vi "Dual_image_synced_pread.vi"() -> ()   [LabVIEW 2013]
uses:
  <vilib>/vision/driver/NI_Vision_Acquisition_Software.lvlib
  <resource>/objmgr/imaqdx.rc
  <resource>/objmgr/daqmx.rc
  <vilib>/DAQmx/configure/timing.llb/DAQmx Timing (Implicit).vi
  <vilib>/DAQmx/create/channels.llb/DAQmx Create Channel (CO-Pulse Generation-Frequency).vi
  <vilib>/DAQmx/create/channels.llb/DAQmx Create Channel (AO-Voltage-Basic).vi
  <vilib>/DAQmx/write.llb/DAQmx Write (Analog DBL 1Chan 1Samp).vi
  <vilib>/DAQmx/create/channels.llb/DAQmx Create Channel (AI-Voltage-Basic).vi
panel:
  in  "File Location":path=path "C:/Users/Public/Documents/Users_2012_2013/Ryan Gergely/ptest/20150925_Accumulator_trials"
  in  "File Name":string="test"
  in  "stop":bool
  out "Pressure Reading":cluster{dbl[], dbl[]}(graph)
  in  "Pressure Offset":dbl
  out "Current Pressure (Psi)":dbl format="%#_4g"
  in  "Sample Frequency (Hz)":dbl=10.0
  in  "Begin Measurement":bool
  in  "Gain 2":dbl(slide)=575.0 min=350.0 max=1000.0 step=1.0 scale=350.0..1000.0
  in  "VR2":dbl(slide)=65.0 min=0.0 max=255.0 step=1.0 scale=0.0..255.0
  in  "VR1":dbl(slide)=60.0 min=0.0 max=255.0 step=1.0 scale=0.0..255.0
  in  "UB2":dbl(slide)=160.0 min=0.0 max=255.0 step=1.0 scale=0.0..255.0
  in  "UB1":dbl(slide)=165.0 min=0.0 max=255.0 step=1.0 scale=0.0..255.0
  in  "Shutter":dbl(slide)=4095.0 min=0.0 max=4095.0 step=1.0 scale=4.095..4095.0 scale format="%#.0f"
  in  "Brightness":dbl(slide)=100.0 min=0.0 max=255.0 step=1.0 scale=0.0..255.0
  in  "Gain":dbl(slide)=600.0 min=350.0 max=1000.0 step=1.0 scale=350.0..1000.0
  in  "Test Description":string="test"
  in  "Storage Directory":path=path "C:/Users/Regen/Desktop/Users/Ryan Gergely/3D_DIC"
  out "Image 2":T1(plugin-control)
  out "Buffer Number 2":u32
  out "Frame Rate 2":dbl
  in  "Camera Name 2":refnum<k21>="cam2" caption="IMAQdx Session"
  in  "Pule Frequency":dbl=2.0 format="%.1f"
  out "Actual Duty Cycle":dbl
  out "Actual Pulse Frequency":dbl
  in  "Stop":bool
  in  "Start Trigger Mode":bool
  out "Frame Rate 1":dbl
  out "Buffer Number 1":u32
  in  "Camera Name 1":refnum<k21>="cam1" caption="IMAQdx Session"
  out "Image":T1(plugin-control)
  # "1) Set Test Description and Storage Directory"
  # "2) Select Cameras"
  # "3) Start VI"
  # "4) Set Frequency and Exposure and White Balance\n(Before Start Trigger)"
  # "5)"
  # "6) Stop When Done"
  # "Exposure Settings - Both Cameras"
  # "White Balance - Camera1"
  # "White Balance - Camera2"
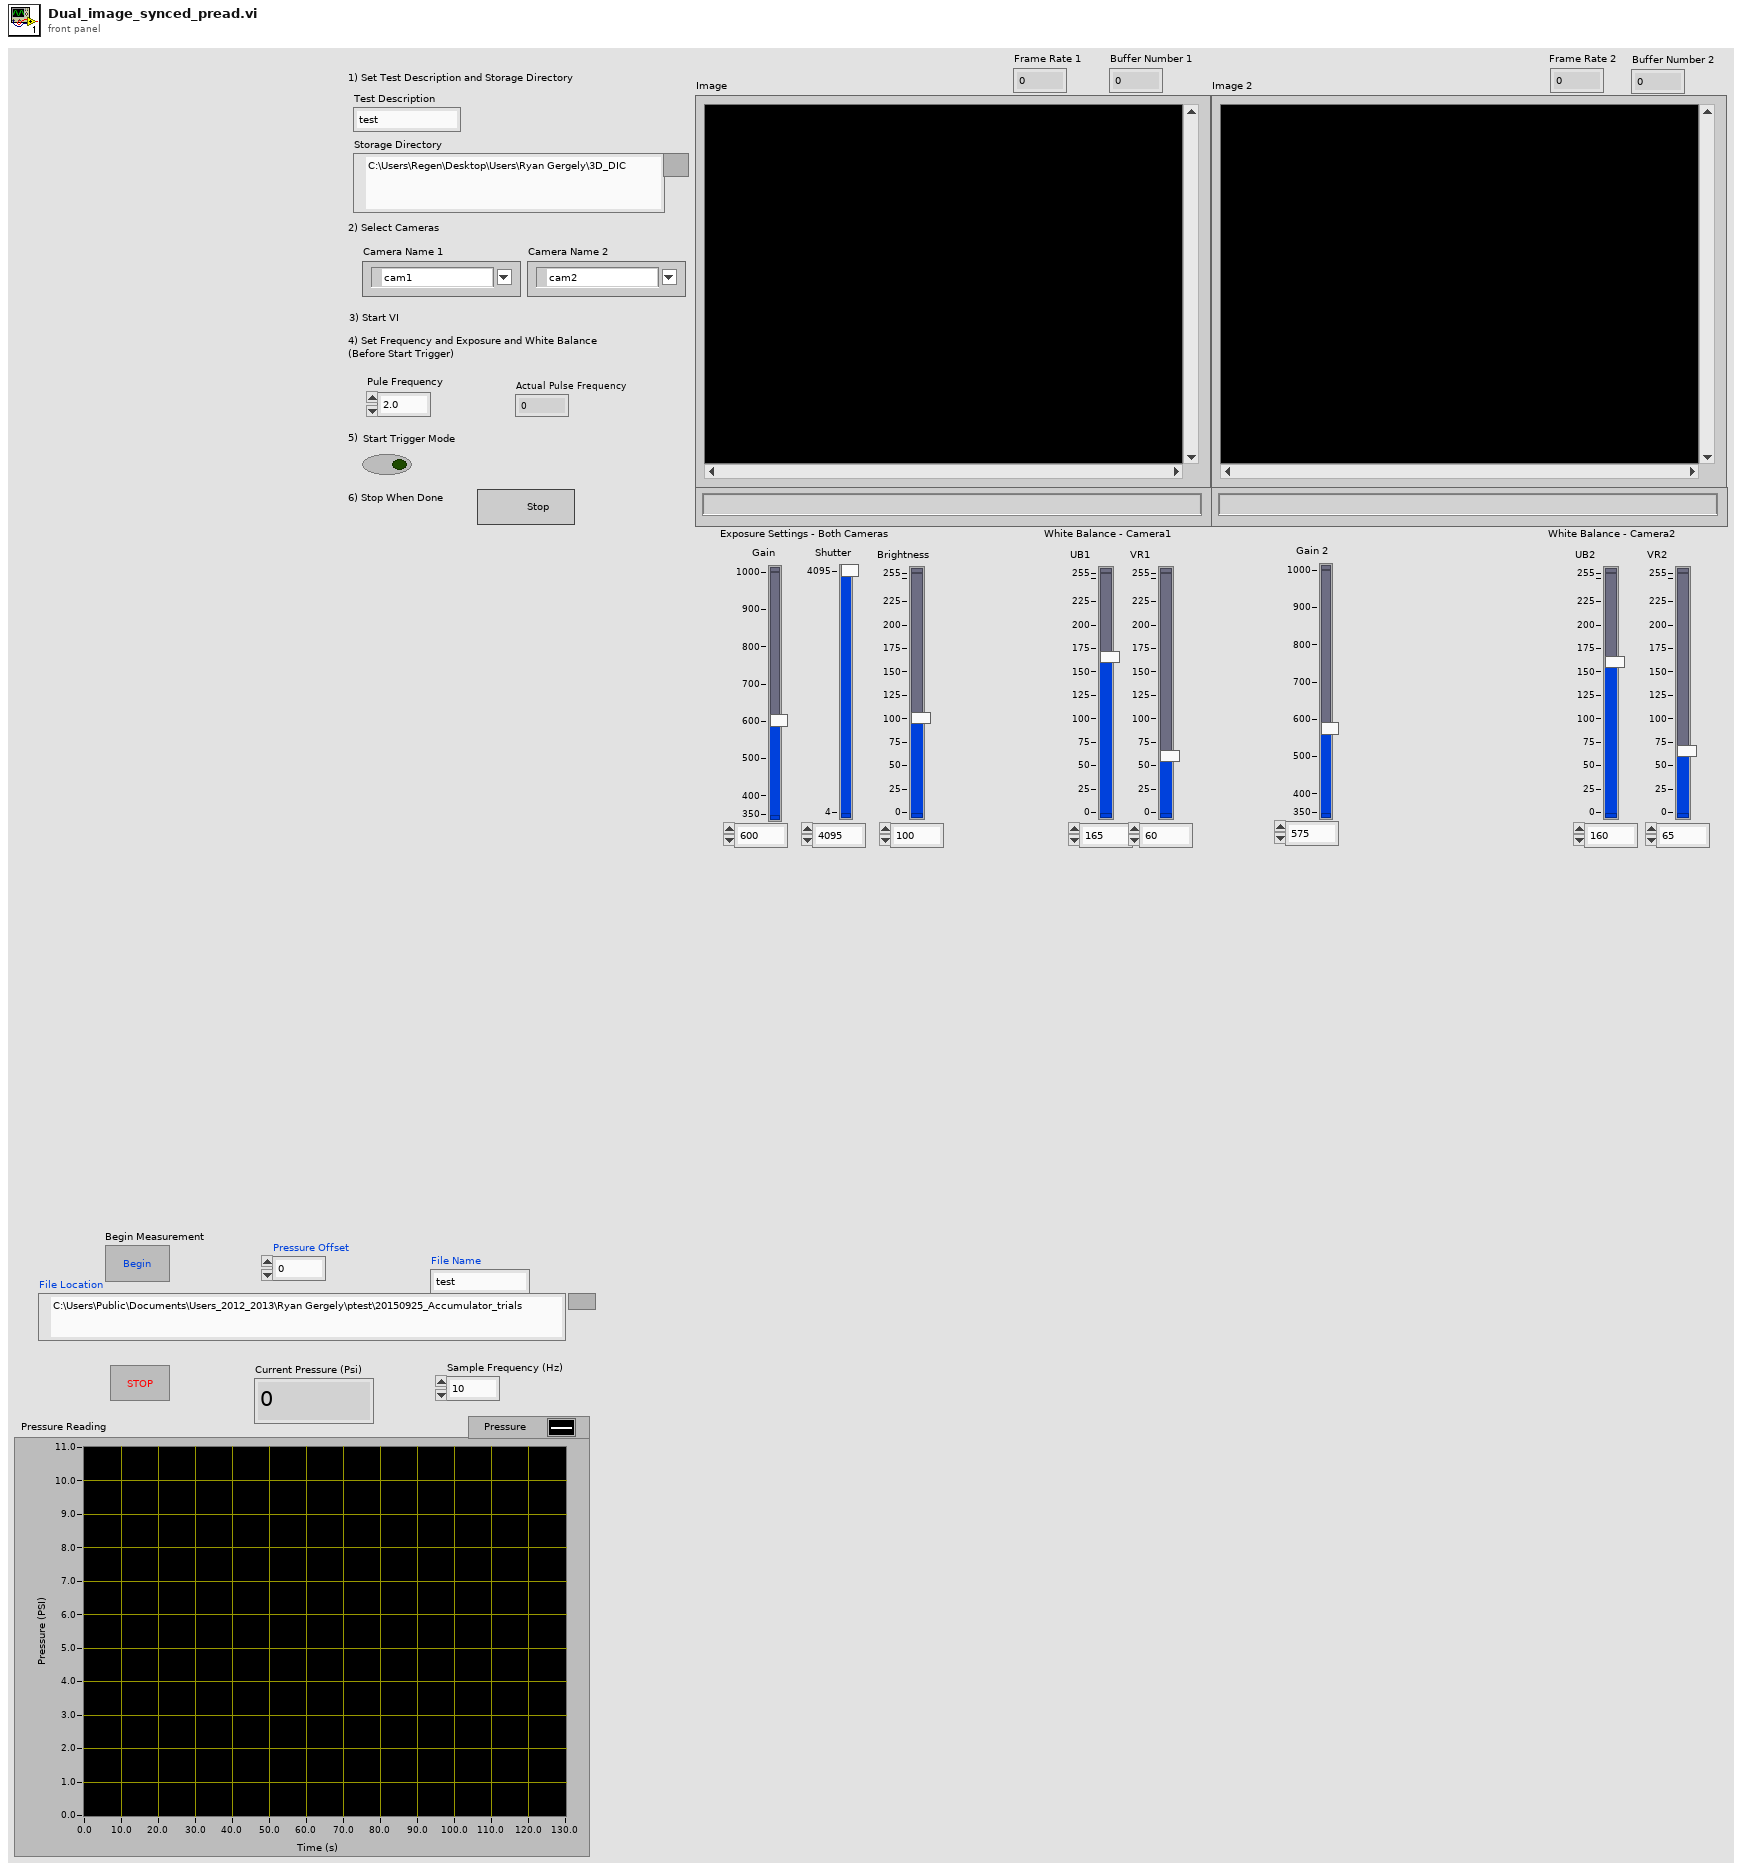
[diagram p1: front panel]
types:
  T1 = typedef "IMAQ Image.ctl" = refnum<image>
  T2 = enum16{"open", "open or create", "create or replace", "create", "open (read only)"}
  T3 = typedef "IMAQdx.ctl" = refnum<k21>
  T4 = cluster{"Trigger Mode":u32, "Trigger Activation":u32, "Timeout (ms)":u32}
  T5 = enum16{"open", "replace", "create", "open or create", "replace or create", "replace or create with confirmation"}
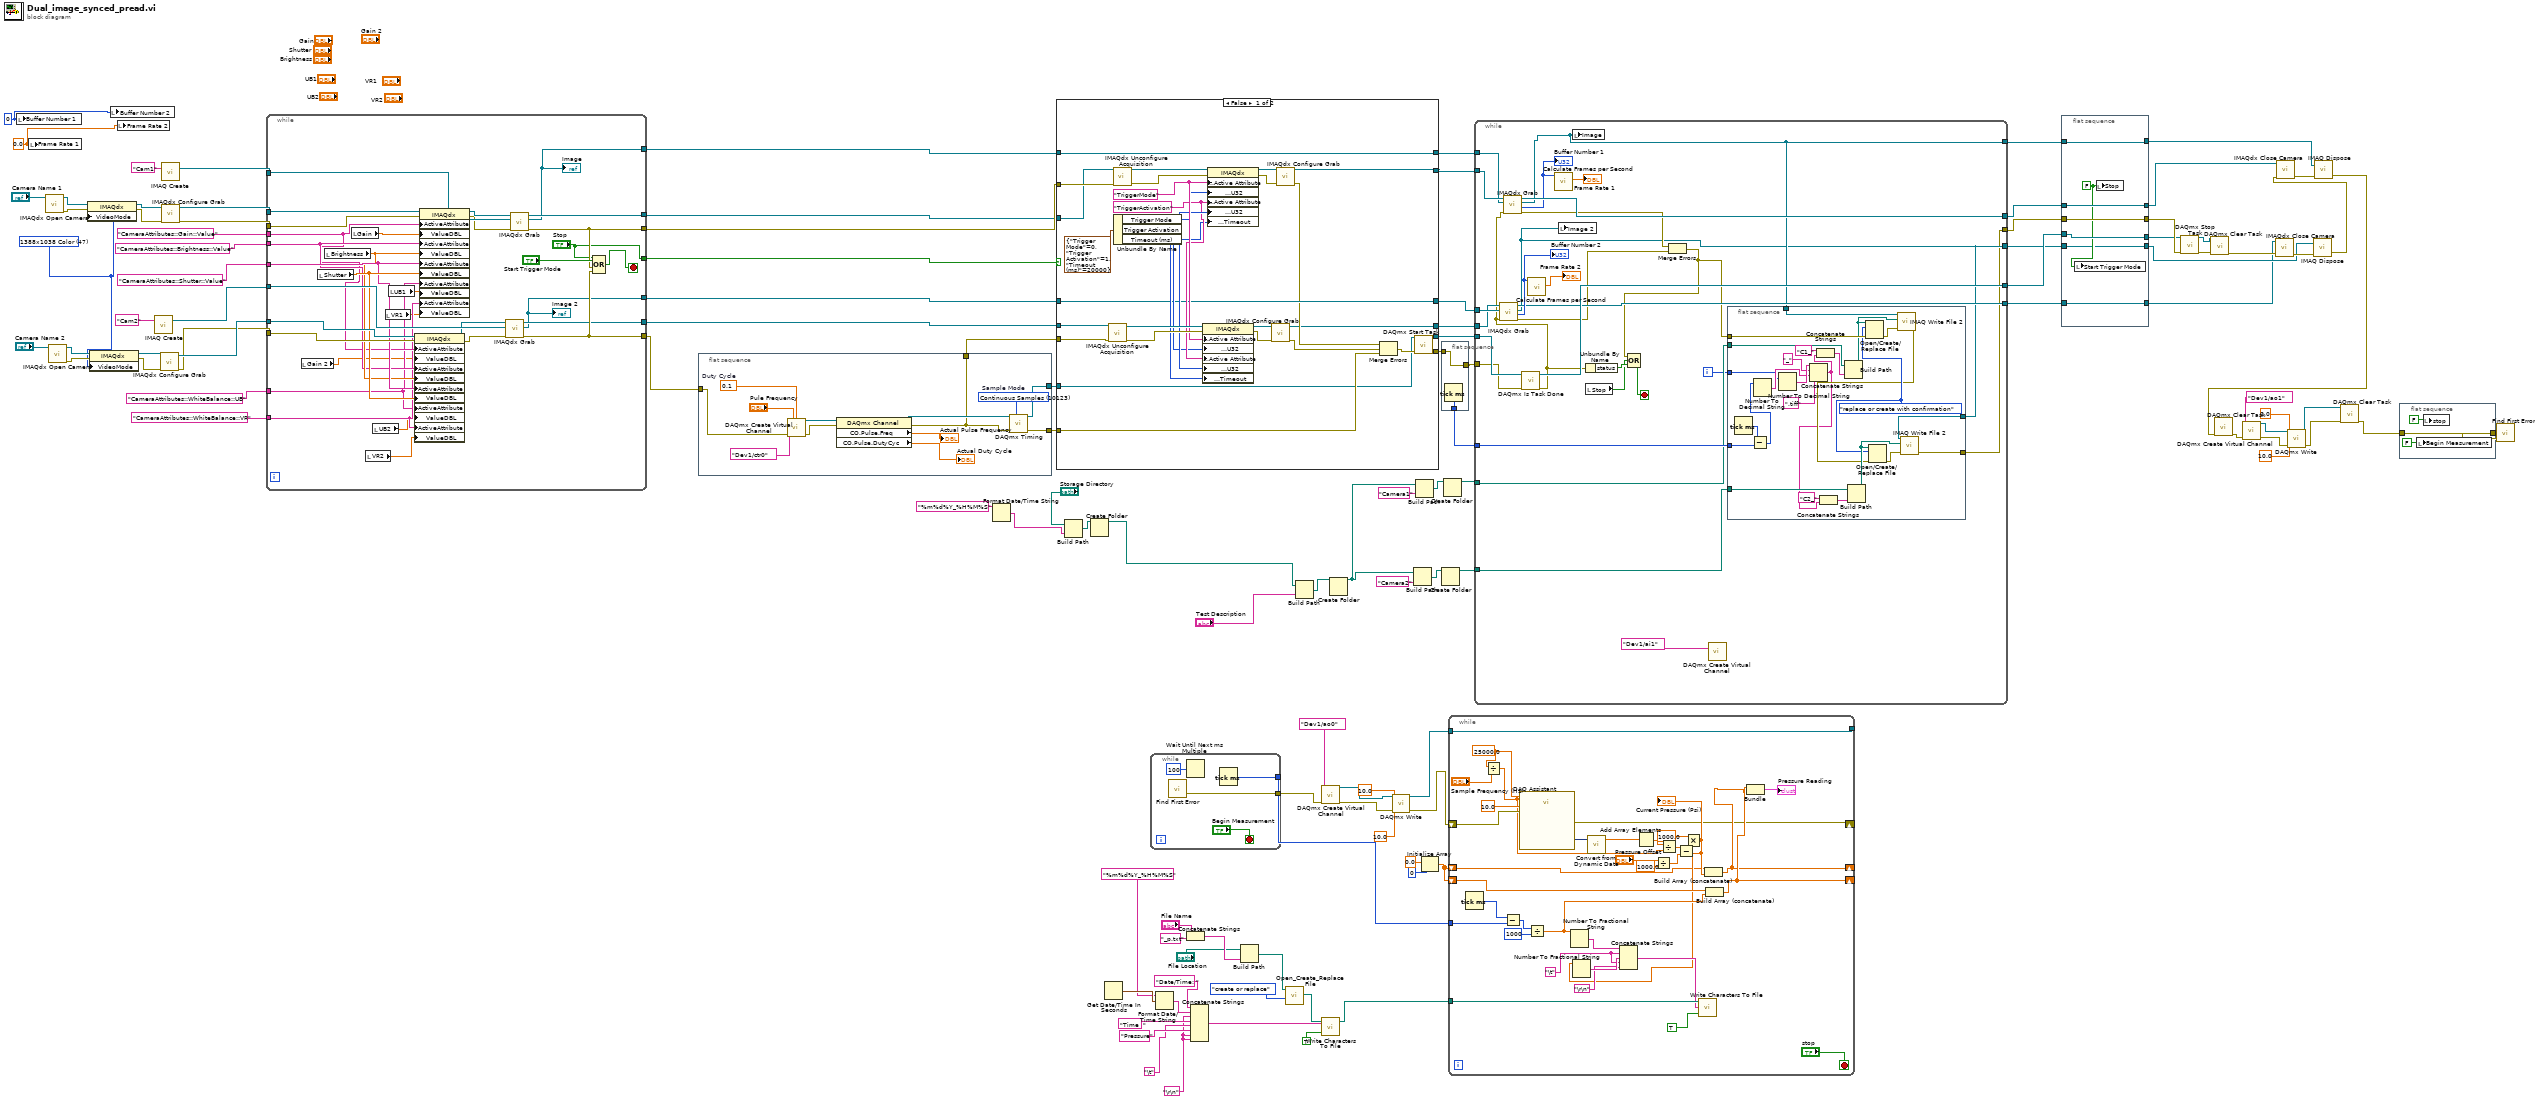
[diagram p0: block diagram]
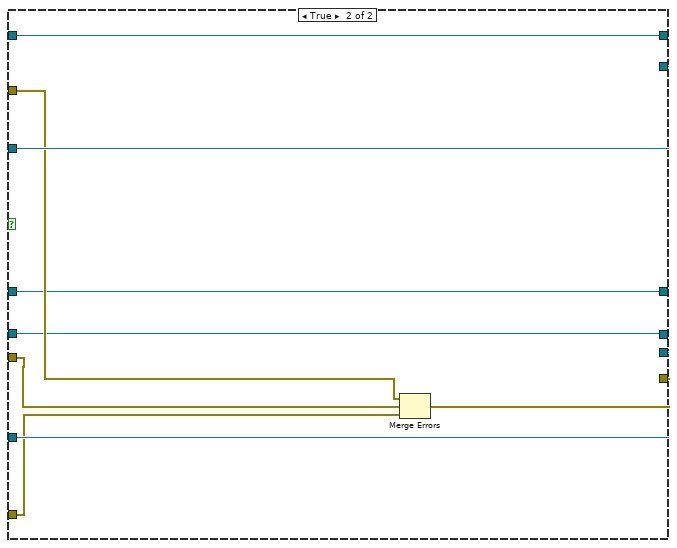
[diagram p2: hidden frame]
diagram:
  w26 = "\r\n"
  w53 = u32 47 items=["320x240 Color"=4, "640x480 Mono8"=9, "640x480 Mono16"=19, "640x480 Color"=14, "800x600 Mono8"=21, "800x600 Mono16"=27, "800x600 Color"=24, "1024x768 Mono8"=30, "1024x768 Mono16"=36, "1024x768 Color"=33, "1280x960 Mono8"=40, "1280x960 Mono16"=46, "1280x960 Color"=43, "1388x1038 Color"=47, "1388x1038 Mono"=48] ("Video Mode")
  w54 = 0.0 ("Frame Rate 1")
  w55 = u32 0 ("Buffer Number 1")
  n1 = local write "Buffer Number 1"(w55) -> ()
  n2 = local write "Frame Rate 1"(w54) -> ()
  n3 = call <vilib>:"IMAQdx Open Camera.vi"("Session In"="Camera Name 1") -> ("error out"=w61:errorcluster, "Session Out"=w63:T3)  [unwired: 2 in, 7 out]
  n4 = call <vilib>:"IMAQdx Open Camera.vi"("Session In"="Camera Name 2") -> ("error out"=w56:errorcluster, "Session Out"=w57:T3)  [unwired: 2 in, 7 out]
  n5 = property class="IMAQdx"(reference=w63, error in=w61, "VideoMode"=w53) -> (reference out=w62:T3, error out=w60:errorcluster)
  n6 = property class="IMAQdx"(reference=w57, error in=w56, "VideoMode"=w53) -> (reference out=w59:T3, error out=w58:errorcluster)
  n7 = local write "Buffer Number 2"(w55) -> ()
  n8 = local write "Frame Rate 2"(w54) -> ()
  n9 = call "IMAQ Create"("Image Name"="Cam2") -> ("New Image"=w50:T1)  [unwired: 3 in, 2 out]
  n10 = call <vilib>:"IMAQdx Configure Grab.vi"("error in"=w58, "Session In"=w59) -> ("error out"=w92:errorcluster, "Session Out"=w93:T3)  [unwired: 8 out]
  n11 = call "IMAQ Create"("Image Name"="Cam1") -> ("New Image"=w103:T1)  [unwired: 3 in, 2 out]
  n12 = call <vilib>:"IMAQdx Configure Grab.vi"("error in"=w60, "Session In"=w62) -> ("error out"=w101:errorcluster, "Session Out"=w102:T3)  [unwired: 8 out]
  n13 = while {
    tunnel: [w149] -> w114
    tunnel: w101 -> [w136]
    tunnel: w102 -> [w138]
    tunnel: [w145] -> w115
    tunnel: w103 -> [w140]
    tunnel: [w148] -> w98
    tunnel: ["Stop"] -> w99
    tunnel: w93 -> [w134]
    tunnel: w92 -> [w133]
    tunnel: [w143] -> w52
    tunnel: [w142] -> w91
    tunnel: [w141] -> w90
    tunnel: w50 -> [w139]
    tunnel: "CameraAttributes::Shutter::Value" ("ActiveAttribute") -> [w129]
    tunnel: "CameraAttributes::Brightness::Value" ("ActiveAttribute") -> [w127]
    tunnel: "CameraAttributes::Gain::Value" ("ActiveAttribute") -> [w125]
    tunnel: "CameraAttributes::WhiteBalance::UB" ("ActiveAttribute") -> [w122]
    tunnel: "CameraAttributes::WhiteBalance::VR" ("ActiveAttribute") -> [w123]
    stop <- w146 stop-if-true
    n14 = local read "Gain 2"() -> (w118:dbl)
    n15 = local read "Shutter"() -> (w130:dbl)
    n16 = local read "Brightness"() -> (w128:dbl)
    n17 = local read "Gain"() -> (w126:dbl)
    n18 = local read "VR2"() -> (w119:dbl)
    n19 = local read "UB2"() -> (w121:dbl)
    n20 = local read "VR1"() -> (w120:dbl)
    n21 = local read "UB1"() -> (w124:dbl)
    n22 = property class="IMAQdx"(reference=w134, error in=w133, "ActiveAttribute"=w125, "ValueDBL"=w118, "ActiveAttribute"=w127, "ValueDBL"=w128, "ActiveAttribute"=w129, "ValueDBL"=w130, "ActiveAttribute"=w122, "ValueDBL"=w121, "ActiveAttribute"=w123, "ValueDBL"=w119) -> (reference out=w131:T3, error out=w132:errorcluster)
    n23 = property class="IMAQdx"(reference=w138, error in=w136, "ActiveAttribute"=w125, "ValueDBL"=w126, "ActiveAttribute"=w127, "ValueDBL"=w128, "ActiveAttribute"=w129, "ValueDBL"=w130, "ActiveAttribute"=w122, "ValueDBL"=w124, "ActiveAttribute"=w123, "ValueDBL"=w120) -> (reference out=w137:T3, error out=w135:errorcluster)
    n24 = call <vilib>:"IMAQdx Grab.vi"("error in"=w132, "Image In"=w139, "Session In"=w131) -> ("error out"=w143:errorcluster, "Image Out"=w141:T1, "Session Out"=w142:T3)  [unwired: 1 in, 5 out]
    "Image 2" <- w141
    n25 = call <vilib>:"IMAQdx Grab.vi"("error in"=w135, "Image In"=w140, "Session In"=w137) -> ("error out"=w145:errorcluster, "Image Out"=w148:T1, "Session Out"=w149:T3)  [unwired: 1 in, 5 out]
    "Image" <- w148
    n26 = Compound Arithmetic op=OR("Stop", "Start Trigger Mode", w145, w143) -> (w146:bool)
  }
  n27 = flat-sequence {
    tunnel: [w153] -> w96
    tunnel: [w152] -> w89
    tunnel: w52 -> [w151]
    tunnel: [w150] -> w51
    frame #0 {
      w160 = 0.1  # Duty Cycle
      w154 = 10123 items=["Finite Samples"=10178, "Continuous Samples"=10123, "Hardware Timed Single Point"=12522]  # Sample Mode
      n28 = call-poly <vilib>:"DAQmx Create Virtual Channel.vi"("frequency"="Pule Frequency", "duty cycle"=w160, "counter"=tag "Dev1/ctr0" ("Counter"), "error in"=w151) -> ("task out"=w156:refnum<k21>, "error out"=w157:errorcluster)  [unwired: 10 in]
      n29 = property class="DAQmx Channel"(reference=w156, error in=w157) -> (reference out=w158:refnum<k21>, error out=w150:errorcluster, "CO.Pulse.Freq"=→"Actual Pulse Frequency":dbl, "CO.Pulse.DutyCyc"=→"Actual Duty Cycle":dbl)
      n30 = call-poly <vilib>:"DAQmx Timing.vi"("task/channels in"=w158, "sample mode"=w154, "error in"=w150) -> ("task out"=w153:refnum<k21>, "error out"=w152:errorcluster)  [unwired: 11 in]
    }
  }
  n31 = Format Date/Time String(time format string (%c)="%m%d%Y_%H%M%S") -> (date/time string=w75:string)  [unwired: 2 in]
  n32 = case shown="False" w99 {
    tunnel: w115 -> [w191 w197]
    tunnel: w114 -> [w190 w200]
    tunnel: [w189 w200] -> w113
    tunnel: [w170 w196] -> w44
    tunnel: [w171 w198] -> w111
    tunnel: w98 -> [w183 w199]
    tunnel: [w183 w199] -> w97
    tunnel: w96 -> [w163 w198]
    tunnel: w51 -> [w174 w195]
    tunnel: w91 -> [w173 w192]
    tunnel: w90 -> [w172 w193]
    tunnel: [w172 w193] -> w88
    tunnel: w89 -> [w166 w194]
    tunnel: [w164 w192] -> w87
    frame False {
      w177 = "TriggerActivation" ("ActiveAttribute")
      w179 = "TriggerMode" ("ActiveAttribute")
      n33 = call <vilib>:"IMAQdx Unconfigure Acquisition.vi"("error in"=w174, "Session In"=w173) -> ("error out"=w181:errorcluster, "Session Out"=w180:T3)  [unwired: 8 out]
      n34 = call <vilib>:"IMAQdx Unconfigure Acquisition.vi"("error in"=w191, "Session In"=w190) -> ("error out"=w186:errorcluster, "Session Out"=w185:T3)  [unwired: 8 out]
      n35 = Unbundle By Name(T4 {"Trigger Mode"=0, "Trigger Activation"=1, "Timeout (ms)"=20000} ("Trigger Parameters")) -> ("Trigger Mode"=w175:u32, "Trigger Activation"=w178:u32, "Timeout (ms)"=w176:u32)
      n36 = property class="IMAQdx"(reference=w180, error in=w181, "Camera Attributes:Active Attribute"=w179, "Camera Attributes:Value:U32"=w175, "Camera Attributes:Active Attribute"=w177, "Camera Attributes:Value:U32"=w178, "Acquisition Attributes:Timeout"=w176) -> (reference out=w182:T3, error out=w169:errorcluster)
      n37 = property class="IMAQdx"(reference=w185, error in=w186, "Camera Attributes:Active Attribute"=w179, "Camera Attributes:Value:U32"=w175, "Camera Attributes:Active Attribute"=w177, "Camera Attributes:Value:U32"=w178, "Acquisition Attributes:Timeout"=w176) -> (reference out=w187:T3, error out=w188:errorcluster)
      n38 = call <vilib>:"IMAQdx Configure Grab.vi"("error in"=w169, "Session In"=w182) -> ("error out"=w167:errorcluster, "Session Out"=w164:T3)  [unwired: 8 out]
      n39 = call <vilib>:"IMAQdx Configure Grab.vi"("error in"=w188, "Session In"=w187) -> ("error out"=w165:errorcluster, "Session Out"=w189:T3)  [unwired: 8 out]
      n40 = Merge Errors(w165, w167, w166) -> (w168:errorcluster)
      n41 = call <vilib>:"DAQmx Start Task.vi"("task/channels in"=w163, "error in"=w168) -> ("task out"=w171:refnum<k21>, "error out"=w170:errorcluster)  [unwired: 12 in]
    }
    frame True {
      n42 = Merge Errors(w197, w195, w194) -> (w196:errorcluster)
    }
  }
  n43 = Build Path(base path="Storage Directory", name or relative path=w75) -> (appended path=w77:path)
  n44 = Create Folder(path (use dialog)=w77) -> (created path=w72:path)  [unwired: 2 in, 2 out]
  n45 = Get Date/Time In Seconds() -> (seconds since 1Jan1904=w25:timestamp)
  n46 = while {
    tunnel: [w203] -> w13
    tunnel: [w202] -> w20
    stop <- "Begin Measurement" stop-if-true
    n47 = call <vilib>:"Find First Error.vi"() -> ("error out"=w203:errorcluster)  [unwired: 4 in, 1 out]
    n48 = Wait Until Next ms Multiple(millisecond multiple=u32 100) -> ()  [unwired: 1 out]
    n49 = Tick Count (ms)() -> (millisecond timer value=w202:u32)
  }
  n50 = Format Date/Time String(time format string (%c)="%m%d%Y_%H%M%S", seconds (now)=w25) -> (date/time string=w33:string)  [unwired: 1 in]
  n51 = Concatenate Strings("File Name", "_p.txt" ("string")) -> (w39:string)
  n52 = Concatenate Strings("Date/Time: ", w33, w26, "Time  ", "\t", "Pressure" ("string"), w26, w26) -> (w34:string)
  n53 = Build Path(base path="File Location", name or relative path=w39) -> (appended path=w30:path)
  n54 = call <vilib>:"Open_Create_Replace File.vi"("function (open:0)"=T2."create or replace", "file path"=w30) -> ("new file path"=w36:path)  [unwired: 6 in, 3 out]
  n55 = Build Path(base path=w72, name or relative path="Test Description") -> (appended path=w71:path)
  n56 = call-poly <vilib>:"DAQmx Create Virtual Channel.vi"("physical channels"=tag "Dev1/ao0", "error in"=w13) -> ("task out"=w14:refnum<k21>, "error out"=w18:errorcluster)  [unwired: 12 in]
  n57 = call <vilib>:"Write Characters To File.vi"("append to file? (new file:F)"=TRUE, "character string"=w34, "file path (dialog if empty)"=w36) -> ("new file path (Not A Path if cancelled)"=w29:path)  [unwired: 2 in]
  n58 = Create Folder(path (use dialog)=w71) -> (created path=w65:path)  [unwired: 2 in, 2 out]
  n59 = call-poly <vilib>:"DAQmx Write.vi"("task/channels in"=w14, "data"=10.0, "timeout"=10.0, "error in"=w18) -> ("task out"=w11:refnum<k21>, "error out"=w12:errorcluster)  [unwired: 9 in, 1 out]
  n60 = Build Path(base path=w65, name or relative path="Camera2") -> (appended path=w66:path)
  n61 = Build Path(base path=w65, name or relative path="Camera1") -> (appended path=w69:path)
  n62 = Initialize Array(0.0 ("element"), 0 ("dimension size")) -> (w22:dbl[])
  n63 = flat-sequence {
    tunnel: w44 -> [w206]
    tunnel: [w206] -> w43
    tunnel: [w205] -> w42
    frame #0 {
      n64 = Tick Count (ms)() -> (millisecond timer value=w205:u32)
    }
  }
  n65 = Create Folder(path (use dialog)=w66) -> (created path=w64:path)  [unwired: 2 in, 2 out]
  n66 = Create Folder(path (use dialog)=w69) -> (created path=w68:path)  [unwired: 2 in, 2 out]
  n67 = while {
    tunnel: w29 -> [w240]
    tunnel: w20 -> [w237]
    shift-right: [w213] -> _
    shift-left: w12 -> [w228]
    shift-right: [w220] -> _
    shift-left: w22 -> [w214]
    shift-right: [w221] -> _
    shift-left: w22 -> [w223]
    tunnel: w11 -> [w219]
    tunnel: [w219] -> _
    stop <- "stop" stop-if-true
    w208 = 25000.0 ("rate")
    w232 = "\t"
    n68 = Tick Count (ms)() -> (millisecond timer value=w238:u32)
    n69 = Divide(x=w208, y="Sample Frequency (Hz)") -> (x/y=w207:dbl)
    n70 = Subtract(x=w238, y=w237) -> (x-y=w236:u32)
    n71 = call "DAQ Assistant"("rate"=w208, "number of samples"=w207, "timeout (s)"=10.0, "error in"=w228) -> ("data"=w229:dynamicdata, "error out"=w213:errorcluster)  [unwired: 13 in, 1 out]
    n72 = Divide(x=w236, y=u32 1000) -> (x/y=w224:dbl)
    n73 = Number To Fractional String(number=w224) -> (F-format string=w234:string)  [unwired: 3 in]
    n74 = call "Convert from Dynamic Data"("Dynamic Data Type"=w229) -> ("Array"=w226:dbl[])  [unwired: 3 in]
    n75 = Add Array Elements(numeric array=w226) -> (sum=w225:dbl)
    n76 = Divide(x="Pressure Offset", y=1000.0) -> (x/y=w210:dbl)
    n77 = Divide(x=w225, y=w207) -> (x/y=w218:dbl)
    n78 = Subtract(x=w218, y=w210) -> (x-y=w216:dbl)
    n79 = Multiply(x=w216, y=1000.0) -> (x*y=w215:dbl)
    "Current Pressure (Psi)" <- w215
    n80 = Number To Fractional String(number=w215) -> (F-format string=w233:string)  [unwired: 3 in]
    n81 = Concatenate Strings(w234, w232, w233, w232, "\r\n") -> (w230:string)
    n82 = call <vilib>:"Write Characters To File.vi"("append to file? (new file:F)"=TRUE, "character string"=w230, "file path (dialog if empty)"=w240) -> ()  [unwired: 2 in, 1 out]
    n83 = Build Array (concatenate)(w214, w215) -> (w220:dbl[])
    n84 = Build Array (concatenate)(w223, w224) -> (w221:dbl[])
    n85 = Bundle(w221, w220) -> (→"Pressure Reading":cluster{dbl[], dbl[]})  [unwired: 1 in]
  }
  n86 = while {
    tunnel: [w269] -> w107
    tunnel: [w247] -> w108
    tunnel: w113 -> [w266]
    tunnel: w97 -> [w265]
    tunnel: [w262] -> w109
    tunnel: w111 -> [w261]
    tunnel: w88 -> [w258]
    tunnel: w87 -> [w257]
    tunnel: w43 -> [w254]
    tunnel: [w251] -> w79
    tunnel: [w250] -> w83
    tunnel: [w253] -> w81
    tunnel: w68 -> [w244]
    tunnel: w64 -> [w252]
    tunnel: w42 -> [w246]
    i -> [w243]
    stop <- w263 stop-if-true
    n87 = call <vilib>:"DAQmx Is Task Done.vi"("task/channels in"=w261, "error in"=w254) -> ("task out"=w262:refnum<k21>, "error out"=w248:errorcluster)  [unwired: 11 in, 1 out]
    n88 = call <vilib>:"IMAQdx Grab.vi"("error in"=w248, "Image In"=w258, "Session In"=w257) -> ("error out"=w249:errorcluster, "Buffer Number Out"=w256:u32, "Image Out"=w250:T1, "Session Out"=w253:T3)  [unwired: 1 in, 4 out]
    "Buffer Number 2" <- w256
    n89 = call <vilib>:"IMAQdx Grab.vi"("error in"=w248, "Image In"=w265, "Session In"=w266) -> ("error out"=w255:errorcluster, "Buffer Number Out"=w267:u32, "Image Out"=w251:T1, "Session Out"=w269:T3)  [unwired: 1 in, 4 out]
    "Buffer Number 1" <- w267
    n90 = call <vilib>:"Calculate Frames per Second.vi"("Buffer Number"=w256) -> ("Processed Frames/s"=→"Frame Rate 2":dbl)  [unwired: 8 in, 2 out]
    n91 = call <vilib>:"Calculate Frames per Second.vi"("Buffer Number"=w267) -> ("Processed Frames/s"=→"Frame Rate 1":dbl)  [unwired: 8 in, 2 out]
    n92 = local write "Image 2"(w250) -> ()
    n93 = local write "Image"(w251) -> ()
    n94 = Unbundle By Name(w248) -> ("status"=w264:bool)
    n95 = local read "Stop"() -> (w260:bool)
    n96 = Merge Errors(w255, w249) -> (w245:errorcluster)
    n97 = Compound Arithmetic op=OR(w245, w260, w264) -> (w263:bool)
    n98 = call-poly <vilib>:"DAQmx Create Virtual Channel.vi"("physical channels"=tag "Dev1/ai1") -> ()  [unwired: 13 in, 2 out]
    n99 = flat-sequence {
      tunnel: w244 -> [w294]
      tunnel: w252 -> [w293]
      tunnel: w251 -> [w292]
      tunnel: w250 -> [w291]
      tunnel: w245 -> [w290]
      tunnel: [w289] -> w247
      tunnel: w246 -> [w282]
      tunnel: w243 -> [w270]
      frame #0 {
        w286 = T5."replace or create with confirmation" ("operation (0:open)")
        n100 = Tick Count (ms)() -> (millisecond timer value=w281:u32)
        n101 = Subtract(x=w281, y=w282) -> (x-y=w280:u32)
        n102 = Number To Decimal String(number=w280) -> (decimal integer string=w273:string)  [unwired: 1 in]
        n103 = Number To Decimal String(number=w270) -> (decimal integer string=w274:string)  [unwired: 1 in]
        n104 = Concatenate Strings(w274, "_" ("string"), w273, ".tiff") -> (w276:string)
        n105 = Concatenate Strings("C1_" ("string"), w276) -> (w279:string)
        n106 = Concatenate Strings("C2_" ("string"), w276) -> (w275:string)
        n107 = Build Path(base path=w294, name or relative path=w279) -> (appended path=w288:path)
        n108 = Build Path(base path=w293, name or relative path=w275) -> (appended path=w287:path)
        n109 = Open/Create/Replace File(file path (use dialog)=w288, error in=w290, operation (0:open)=w286) -> (error out=w285:errorcluster)  [unwired: 3 in, 2 out]
        n110 = call-poly "IMAQ Write File 2"("error in (no error)"=w285, "File Path"=w288, "Image"=w292) -> ("error out"=w283:errorcluster)  [unwired: 7 in, 1 out]
        n111 = Open/Create/Replace File(file path (use dialog)=w287, error in=w283, operation (0:open)=w286) -> (error out=w284:errorcluster)  [unwired: 3 in, 2 out]
        n112 = call-poly "IMAQ Write File 2"("error in (no error)"=w284, "File Path"=w287, "Image"=w291) -> ("error out"=w289:errorcluster)  [unwired: 7 in, 1 out]
      }
    }
  }
  n113 = flat-sequence {
    tunnel: w109 -> [w299]
    tunnel: w108 -> [w300]
    tunnel: w107 -> [w301]
    tunnel: [w301] -> w106
    tunnel: [w300] -> w105
    tunnel: [w299] -> w104
    tunnel: [w297] -> w82
    tunnel: w83 -> [w297]
    tunnel: w81 -> [w296]
    tunnel: [w296] -> w80
    tunnel: w79 -> [w295]
    tunnel: [w295] -> w78
    frame #0 {
      w298 = FALSE ("Stop")
      n114 = local write "Start Trigger Mode"(w298) -> ()
      n115 = local write "Stop"(w298) -> ()
    }
  }
  n116 = call <vilib>:"DAQmx Stop Task.vi"("task/channels in"=w104, "error in"=w105) -> ("task out"=w110:refnum<k21>, "error out"=w112:errorcluster)  [unwired: 12 in]
  n117 = call <vilib>:"DAQmx Clear Task.vi"("task in"=w110, "error in"=w112) -> ("error out"=w84:errorcluster)  [unwired: 13 in]
  n118 = call <vilib>:"IMAQdx Close Camera.vi"("error in"=w84, "Session In"=w80) -> ("error out"=w86:errorcluster)  [unwired: 9 out]
  n119 = call "IMAQ Dispose"("Image"=w82, "error in (no error)"=w86) -> ("error out"=w85:errorcluster)  [unwired: 4 in]
  n120 = call <vilib>:"IMAQdx Close Camera.vi"("error in"=w85, "Session In"=w106) -> ("error out"=w117:errorcluster)  [unwired: 9 out]
  n121 = call "IMAQ Dispose"("Image"=w78, "error in (no error)"=w117) -> ("error out"=w1:errorcluster)  [unwired: 4 in]
  n122 = call <vilib>:"DAQmx Clear Task.vi"("error in"=w1) -> ("error out"=w9:errorcluster)  [unwired: 14 in]
  n123 = call-poly <vilib>:"DAQmx Create Virtual Channel.vi"("physical channels"=tag "Dev1/ao1", "error in"=w9) -> ("task out"=w4:refnum<k21>, "error out"=w10:errorcluster)  [unwired: 12 in]
  n124 = call-poly <vilib>:"DAQmx Write.vi"("task/channels in"=w4, "data"=0.0, "timeout"=10.0, "error in"=w10) -> ("task out"=w3:refnum<k21>, "error out"=w8:errorcluster)  [unwired: 9 in, 1 out]
  n125 = call <vilib>:"DAQmx Clear Task.vi"("task in"=w3, "error in"=w8) -> ("error out"=w2:errorcluster)  [unwired: 13 in]
  n126 = flat-sequence {
    tunnel: w2 -> [w304]
    tunnel: [w304] -> w21
    frame #0 {
      n127 = local write "Begin Measurement"(FALSE ("Begin Measurement")) -> ()
      n128 = local write "stop"(FALSE ("stop")) -> ()
    }
  }
  n129 = call <vilib>:"Find First Error.vi"("error in (no error)"=w21) -> ()  [unwired: 3 in, 2 out]
